vi "Omni-teste-Fast-delay.vi"() -> ()   [LabVIEW 2014]
doc: "André Romero - 2016\nandretec@ifsc.usp.br"
panel:
  out "Waveform Chart":u32(graph)=100
  out "delay":u32=100
  in  "stop":bool
  out "XY Graph":T1(graph)
  out "Length":i32=2048
  in  "Correct Electrical Dark":bool=TRUE
  in  "Integration Time (ms)":i32=100
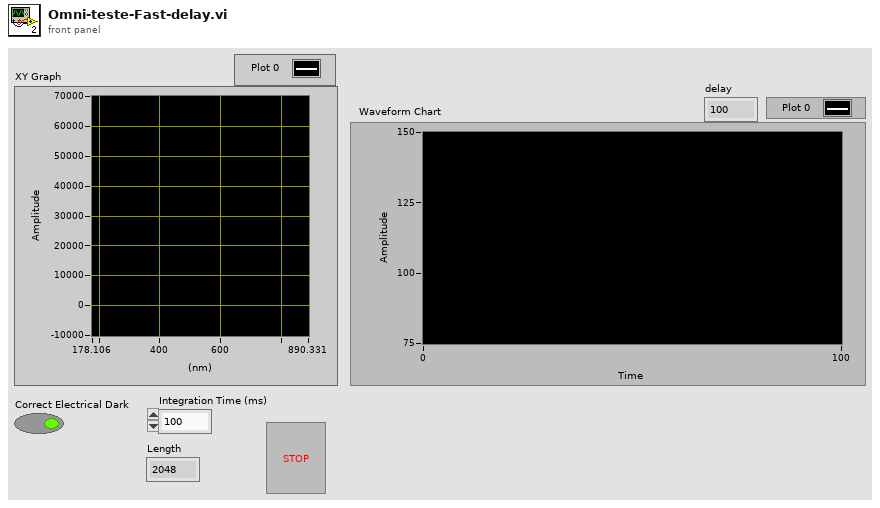
[diagram p1: front panel]
types:
  T1 = cluster{"WL Values":dbl[], "Spectrum Values":dbl[]}
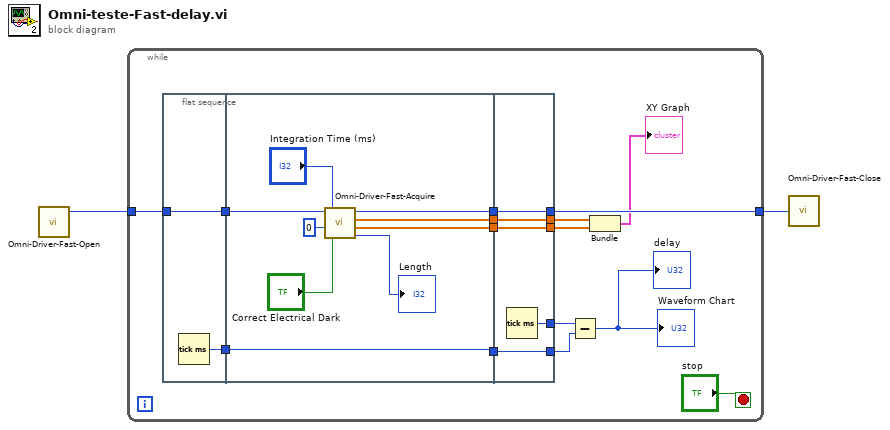
[diagram p0: block diagram]
diagram:
  n1 = call "Omni-Driver-Fast-Open.vi"() -> ("Wrapper Out"=w2:u32)  [unwired: 4 in, 1 out]
  n2 = while {
    tunnel: w2 -> [w17]
    tunnel: [w16] -> w1
    stop <- "stop" stop-if-true
    n3 = flat-sequence {
      tunnel: w17 -> [w19]
      tunnel: [w19] -> w11
      tunnel: [w18] -> w5
      tunnel: w11 -> [w28]
      tunnel: [w27] -> w10
      tunnel: [w23] -> w9
      tunnel: [w22] -> w8
      tunnel: [w20] -> w6
      tunnel: w5 -> [w20]
      tunnel: [w31] -> w13
      tunnel: [w32] -> w14
      tunnel: [w33] -> w16
      tunnel: w10 -> [w33]
      tunnel: w9 -> [w32]
      tunnel: w8 -> [w31]
      tunnel: [w30] -> w7
      tunnel: w6 -> [w29]
      tunnel: [w29] -> w4
      frame #0 {
        n4 = Tick Count (ms)() -> (millisecond timer value=w18:u32)
      }
      frame #1 {
        n5 = call "Omni-Driver-Fast-Acquire.vi"("Correct Electrical Dark"="Correct Electrical Dark", "Spectrometer number"=0, "Integration Time (ms)"="Integration Time (ms)", "Wrapper"=w28) -> ("Length"=→"Length":i32, "Spectrum Values"=w22:dbl[], "WL Values"=w23:dbl[], "Wrapper Out"=w27:u32)
      }
      frame #2 {
        n6 = Tick Count (ms)() -> (millisecond timer value=w30:u32)
      }
    }
    n7 = Subtract(x=w7, y=w4) -> (x-y=→"delay" →"Waveform Chart":u32)
    n8 = Bundle("WL Values"=w14, "Spectrum Values"=w13) -> (→"XY Graph":T1)  [unwired: 1 in]
  }
  n9 = call "Omni-Driver-Fast-Close.vi"("Wrapper In"=w1) -> ()  [unwired: 1 in]
